vi "Close.vi"(8 "error in":errorcluster, 11 "Combo Box in":refnum<class "Combo Box.lvclass">) -> (0 "error out":errorcluster, 3 "Combo Box out":refnum<class "Combo Box.lvclass">)   [LabVIEW 2023, in "SourceGrid.lvlib" / "Combo Box.lvclass"]
uses:
  Combo Box.lvclass
  Combo Box.lvclass/Combo Box.ctl
  D:/git/Sourcegrid-LabVIEW/dll/SourceGrid.dll
  dll/SourceGrid.dll
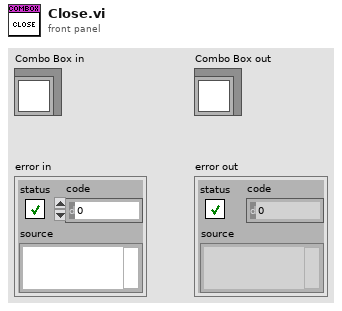
[diagram p1: front panel]
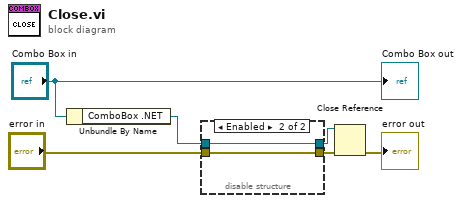
[diagram p0: block diagram]
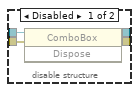
[diagram p2: hidden frame]
diagram:
  n1 = Unbundle By Name("Combo Box in") -> ("ComboBox .NET"=w2:refnum<k24>)
  n2 = disable-structure shown="Enabled" {
    disable-tunnel: "error in" -> [w10 w12]
    disable-tunnel: [w9 w12] -> w3
    disable-tunnel: w2 -> [w8 w11]
    disable-tunnel: [w7 w11] -> w1
    frame Disabled {
      n3 = invoke class="ComboBox" method="Dispose"(reference=w8, error in=w10) -> (reference out=w7:refnum<k24>, error out=w9:errorcluster)  [unwired: 1 in, 1 out]
    }
    frame Enabled {
    }
  }
  n4 = Close Reference(reference=w1, error in (no error)=w3) -> (error out=→"error out":errorcluster)
  "Combo Box out" <- "Combo Box in"
